vi "Intake Wheels Controller.vi"(8 "error in":errorcluster) -> ()   [LabVIEW 2017]
doc: "This VI executes continuously carrying out the current operation and responding to updates or new operations. It will often contain the timing or control code that is difficult to place directly in TeleOp. This VI generally opens all sensors and motors and isolates the rest of the robot code from knowing how the operations are carried out."
uses:
  <vilib>/Rock Robotics/WPI/Framework/Completion Status.ctl
  Intake Wheels Setpoints.ctl
  Intake Wheels Operations.ctl
  <vilib>/Rock Robotics/WPI/Solenoid/WPI_SolenoidValue.ctl
  <vilib>/Rock Robotics/WPI/Solenoid/WPI_SolenoidChannel.ctl
  Users/Public/Documents/Cross The Road Electronics/Phoenix-LabVIEW/Motor Controller/Controls/CTRE_Phoenix_MotorControl_ControlMode.ctl
  <vilib>/Rock Robotics/WPI/ThirdParty/Phoenix-LabVIEW/Motor Controller/Controls/CTRE_Phoenix_MotorControl_NeutralMode.ctl
  <vilib>/Rock Robotics/WPI/Solenoid/WPI_SolenoidOpenSingle.vi
  <vilib>/Rock Robotics/WPI/Solenoid/WPI_SolenoidSetEnum.vi
  <vilib>/Rock Robotics/Network Tables/NT Write Boolean.vi
panel:
  in  "Interactive Values":T1
  out "Current\nCmd":string
  in  "Buttons":cluster{"Execute Cmd":bool, "Abort Cmd":bool}
  out "Command Timing":cluster{"Start Time (ms)":u32, "Iterations":i32}
  out "Status":T3
  # "Tip: It may be helpful to observe inputs and sensor values.\nYou may also want to display tuning or debugging controls."
  # "Interactive Command: You may fill in the settings for a command\nand schedule it with the Execute button. You can observe and abort\nany command while fine tuning the code for the controller."
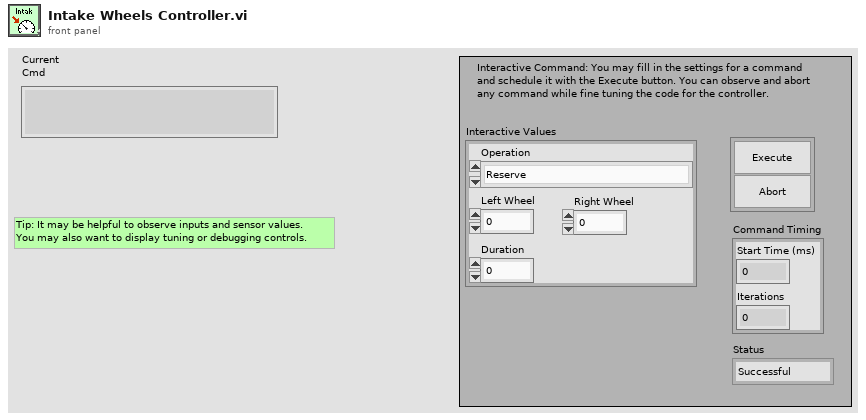
[diagram p1: front panel]
types:
  T1 = typedef "Intake Wheels Setpoints.ctl" = cluster{"Operation":T2, "Left Wheel":dbl, "Duration":dbl, "Right Wheel":dbl}
  T2 = typedef "Intake Wheels Operations.ctl" = enum16{"Reserve", "Read Current", "Immediate", "Intake Open", "Intake Close", "Wheels On"}
  T3 = typedef "Completion Status.ctl" = enum16{"Successful", "Aborted", "Incomplete"}
  T4 = typedef "CTRE_Phoenix_MotorControl_NeutralMode.ctl" = enum8{"EEPROMSetting", "Override to Coast", "Override to Brake"}
  T5 = typedef "CTRE_Phoenix_MotorControl_ControlMode.ctl" = u16
  T6 = typedef "WPI_SolenoidChannel.ctl" = enum8{"Solenoid 0", "Solenoid 1", "Solenoid 2", "Solenoid 3", "Solenoid 4", "Solenoid 5", "Solenoid 6", "Solenoid 7", "Invalid"}
  T7 = typedef "WPI_SolenoidValue.ctl" = enum16{"Off", "On", "Forward", "Reverse"}
  T8 = typedef "WPI_SolenoidDevRef.ctl" = cluster{"DevStatus":errorcluster, "Pneumatics Control Module":u8, "Forward Solenoid Channel":T6, "Reverse Solenoid Channel":T6}
  T9 = typedef "WPI_MotorControlDeviceRef.ctl" = cluster{"DeviceStatus":errorcluster, "Type":T10, "PWM":cluster{"PWM Channel":T11, "DeadBand":T12}, "CAN":cluster{"Device Number":u8, "SetOutput VI Ref":variant, "GetOutput VI Ref":variant, "Enable VI Ref":variant, "Disable VI Ref":variant, "Data":variant}, "Invert":bool, "DIO PWM":cluster{"PWM \"Enable\" Channel":T11, "DIOChannel":T13, "PWM Rate":dbl}}
  T10 = typedef "WPI_MotorControlType.ctl" = enum16{"PWM", "CAN", "DIO PWM"}
  T11 = typedef "FPGA_DIOPWMChannel.ctl" = enum8{"PWM 0", "PWM 1", "PWM 2", "PWM 3", "PWM 4", "PWM 5", "PWM 6", "PWM 7", "PWM 8", "PWM 9", "PWM MXP 0", "PWM MXP 1", "PWM MXP 2", "PWM MXP 3", "PWM MXP 4", "PWM MXP 5", "PWM MXP 6", "PWM MXP 7", "PWM MXP 8", "PWM MXP 9", "Invalid"}
  T12 = typedef "WPI_PWMDeadband.ctl" = cluster{"Name":string, "maxPositivePwm":i32, "minPositivePwm":i32, "centerPwm":i32, "maxNegativePwm":i32, "minNegativePwm":i32, "angularRange":u16}
  T13 = typedef "FPGA_DIOChannel.ctl" = enum8{"DIO 0", "DIO 1", "DIO 2", "DIO 3", "DIO 4", "DIO 5", "DIO 6", "DIO 7", "DIO 8", "DIO 9", "DIO MXP 0", "DIO MXP 1", "DIO MXP 2", "DIO MXP 3", "DIO MXP 4", "DIO MXP 5", "DIO MXP 6", "DIO MXP 7", "DIO MXP 8", "DIO MXP 9", "DIO MXP 10", "DIO MXP 11", "DIO MXP 12", "DIO MXP 13", "DIO MXP 14", "DIO MXP 15", "SPI Port CS1", "SPI Port CS2", "SPI Port CS3", "SPI Port MISO", "SPI Port MOSI", "Invalid"}
  T14 = typedef "Command Status Info.ctl" = cluster{"Name":string, "Status":T3, "notifier out":T15}
  T15 = typedef "Completion Notifier.ctl" = refnum<notifier>
  T16 = cluster{"Current Command":T1, "Command Timing":cluster{"Start Time (ms)":u32, "Iterations":i32}, "Command Arguments":cluster{"Command Info":T14, "Description":string, "Default Command":T1, "queue out":refnum<queue>, "Subsystem Name":string}}
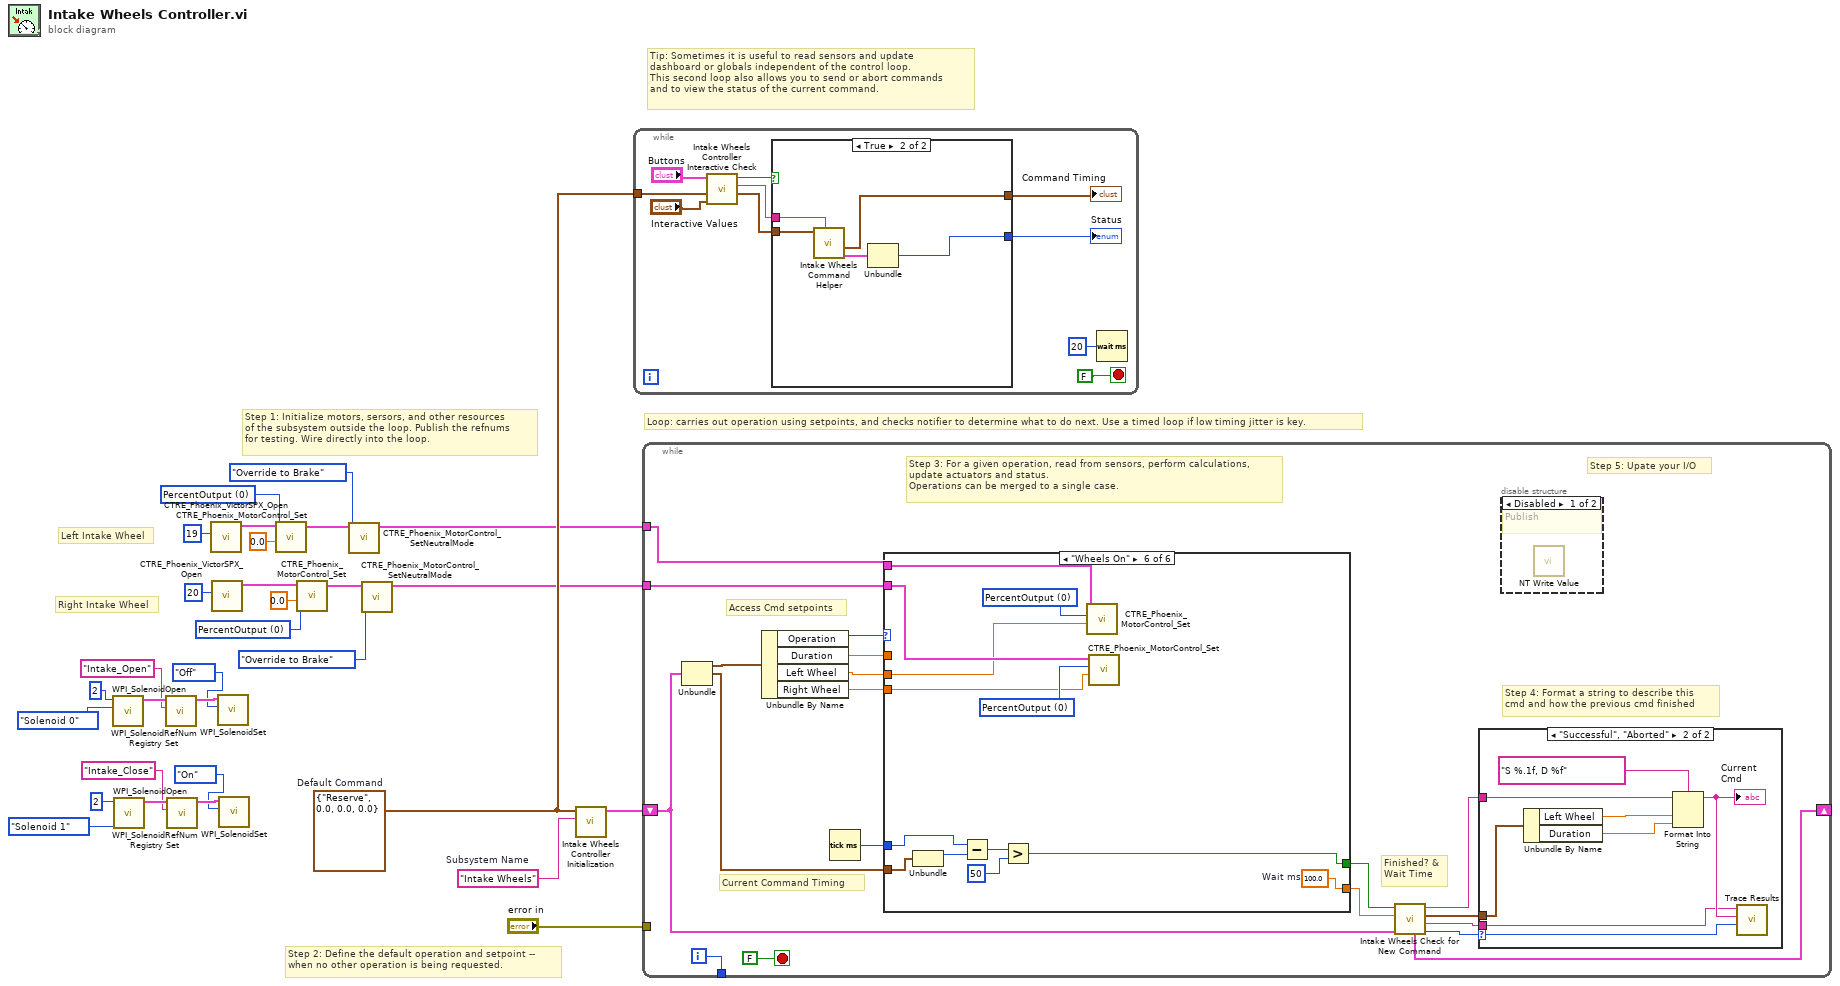
[diagram p0: block diagram]
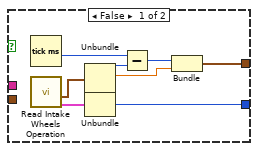
[diagram p2: hidden frame]
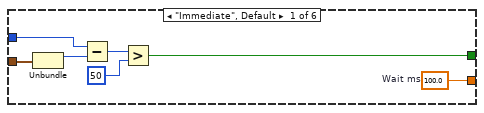
[diagram p5: hidden frame]
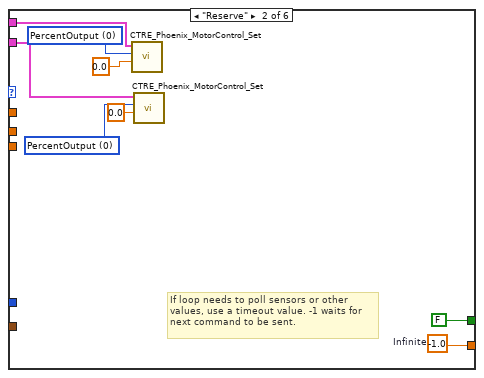
[diagram p6: hidden frame]
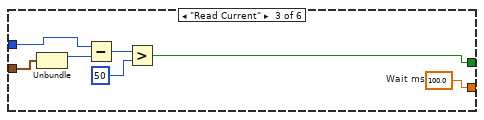
[diagram p7: hidden frame]
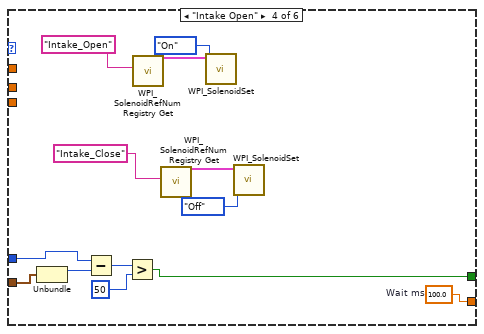
[diagram p8: hidden frame]
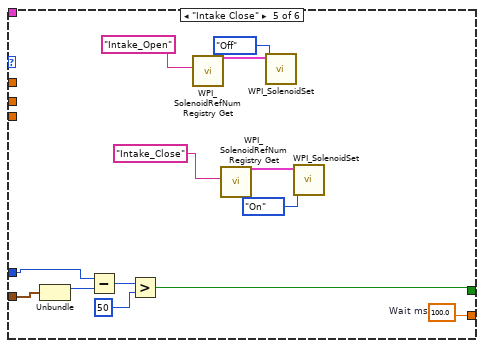
[diagram p9: hidden frame]
diagram:
  w10 = T5 0 items=["PercentOutput"=0, "Position"=1, "Velocity"=2, "Current"=3, "Follower"=5, "MotionProfile"=6, "MotionMagic"=7, "MotionMagicArc"=8, "MotionProfileArc"=10, "Disabled"=15] ("Control Mode")
  w11 = T5 0 items=["PercentOutput"=0, "Position"=1, "Velocity"=2, "Current"=3, "Follower"=5, "MotionProfile"=6, "MotionMagic"=7, "MotionMagicArc"=8, "MotionProfileArc"=10, "Disabled"=15] ("Control Mode")
  w27 = T1 {"Operation"=enum."Reserve", "Left Wheel"=0.0, "Duration"=0.0, "Right Wheel"=0.0}  # Default Command
  w28 = "Intake Wheels"  # Subsystem Name
  # "Right Intake Wheel"
  # "Left Intake Wheel"
  # "Tip: Sometimes it is useful to read sensors and update\ndashboard or globals independent of the control loop.\nThis second loop also allows you to send or abort commands\nand to view the status of the current command."
  # "Step 2: Define the default operation and setpoint --\nwhen no other operation is being requested."
  # "Step 1: Initialize motors, sersors, and other resources\nof the subsystem outside the loop. Publish the refnums\nfor testing. Wire directly into the loop."
  # "Loop: carries out operation using setpoints, and checks notifier to determine what to do next. Use a timed loop if low timing jitter is key."
  n1 = call-poly <vilib>:"WPI_SolenoidOpen.vi"("Solenoid Channel"=WPI_SolenoidChannel."Solenoid 0", "Pneumatics Control Module (0)"=u8 2) -> ("SolenoidDevRef"=w26:T8)  [unwired: 8 in, 1 out]
  n2 = call-poly <vilib>:"WPI_SolenoidOpen.vi"("Solenoid Channel"=WPI_SolenoidChannel."Solenoid 1", "Pneumatics Control Module (0)"=u8 2) -> ("SolenoidDevRef"=w21:T8)  [unwired: 8 in, 1 out]
  n3 = call <vilib>:"WPI_SolenoidRefNum Registry Set.vi"("refnum name"="Intake_Open", "SolenoidDevRef"=w26) -> ("SolenoidDevRef"=w25:T8)  [unwired: 8 in, 1 out]
  n4 = call <vilib>:"WPI_SolenoidRefNum Registry Set.vi"("refnum name"="Intake_Close", "SolenoidDevRef"=w21) -> ("SolenoidDevRef"=w20:T8)  [unwired: 8 in, 1 out]
  n5 = call <vilib>:"CTRE_Phoenix_VictorSPX_Open.vi"("Device Number"=u8 19) -> ("CAN Talon SRX Ref"=w12:T9)  [unwired: 9 in, 1 out]
  n6 = call <vilib>:"CTRE_Phoenix_VictorSPX_Open.vi"("Device Number"=u8 20) -> ("CAN Talon SRX Ref"=w9:T9)  [unwired: 9 in, 1 out]
  n7 = call-poly <vilib>:"WPI_SolenoidSet.vi"("Value"=WPI_SolenoidValue."Off", "SolenoidDevRef"=w25) -> ()  [unwired: 8 in, 2 out]
  n8 = call-poly <vilib>:"WPI_SolenoidSet.vi"("Value"=WPI_SolenoidValue."On", "SolenoidDevRef"=w20) -> ()  [unwired: 8 in, 2 out]
  n9 = call <vilib>:"CTRE_Phoenix_MotorControl_Set.vi"("Output"=0.0, "Control Mode"=w11, "PhoenixMotorControlDevRef"=w12) -> ("PhoenixMotorControlDevRef"=w8:T9)  [unwired: 7 in, 1 out]
  n10 = call <vilib>:"CTRE_Phoenix_MotorControl_Set.vi"("Output"=0.0, "Control Mode"=w10, "PhoenixMotorControlDevRef"=w9) -> ("PhoenixMotorControlDevRef"=w6:T9)  [unwired: 7 in, 1 out]
  n11 = call <vilib>:"CTRE_Phoenix_MotorControl_SetNeutralMode.vi"("Motor Control Neutral Mode"=CTRE_Phoenix_MotorControl_NeutralMode."Override to Brake", "PhoenixMotorControlDevRef"=w8) -> ("PhoenixMotorControlDevRef"=w2:T9)  [unwired: 8 in, 1 out]
  n12 = call <vilib>:"CTRE_Phoenix_MotorControl_SetNeutralMode.vi"("Motor Control Neutral Mode"=CTRE_Phoenix_MotorControl_NeutralMode."Override to Brake", "PhoenixMotorControlDevRef"=w6) -> ("PhoenixMotorControlDevRef"=w1:T9)  [unwired: 8 in, 1 out]
  n13 = call "Intake Wheels Controller Initialization.vi"("Subsystem Name"=w28, "Default Command"=w27) -> ("Current Command"=w29:T16)  [unwired: 9 in]
  n14 = while {
    tunnel: w27 -> [w37]
    stop <- FALSE stop-if-true
    n15 = call "Intake Wheels Controller Interactive Check.vi"("Interactive Command in"="Interactive Values", "Default Command"=w37, "Buttons"="Buttons") -> ("Interactive Command out"=w34:T1, "Trace String"=w35:string, "Schedule"=w36:bool)  [unwired: 6 in]
    n16 = case shown="True" w36 {
      tunnel: [w48 w53] -> w33
      tunnel: w34 -> [_ w51]
      tunnel: [w44 w49] -> w32
      tunnel: w35 -> [_ w52]
      frame False {
        n17 = Tick Count (ms)() -> (millisecond timer value=w43:u32)
        n18 = call "Read Intake Wheels Operation.vi"() -> ("Command Info"=w41:T14, "SubSystem Data"=w42:T1)  [unwired: 9 in, 1 out]
        n19 = Unbundle(w42) -> ("Operation"=w47:T2, "Left Wheel"=w45:dbl)  [unwired: 2 out]
        n20 = Unbundle(w41) -> ("Status"=w48:T3)  [unwired: 2 out]
        n21 = Subtract(x=w43, y=w47) -> (x-y=w46:u32)
        n22 = Bundle(w46, "Left Wheel"=w45) -> (w44:cluster{u32, "Left Wheel":dbl})  [unwired: 1 in]
      }
      frame True {
        n23 = call "Intake Wheels Command Helper.vi"("Description"=w52, "SubSystem Data"=w51) -> ("Command Info Out"=w50:T14, "Command Timing"=w49:cluster{"Start Time (ms)":u32, "Iterations":i32})  [unwired: 7 in, 1 out]
        n24 = Unbundle(w50) -> ("Status"=w53:T3)  [unwired: 2 out]
      }
    }
    "Status" <- w33
    "Command Timing" <- w32
    n25 = Wait (ms)(milliseconds to wait=u32 20) -> ()  [unwired: 1 out]
  }
  n26 = while {
    shift-right: [w64] -> _
    shift-left: w29 -> [w57]
    tunnel: [w71] -> _
    tunnel: "error in" -> [_]
    tunnel: w2 -> [w56]
    tunnel: w1 -> [w55]
    i -> [w71]
    stop <- FALSE stop-if-true
    # "Step 5: Upate your I/O"
    # "Step 4: Format a string to describe this\ncmd and how the previous cmd finished"
    # "Current Command Timing"
    # "Access Cmd setpoints"
    # "Finished? &\nWait Time"
    # "Step 3: For a given operation, read from sensors, perform calculations,\nupdate actuators and status.\nOperations can be merged to a single case."
    n27 = Unbundle(w57) -> ("Current Command"=w70:T1, "Command Timing"=w66:cluster{"Start Time (ms)":u32, "Iterations":i32})  [unwired: 1 out]
    n28 = Unbundle By Name(w70) -> ("Operation"=w69:T2, "Duration"=w68:dbl, "Left Wheel"=w65:dbl, "Right Wheel"=w54:dbl)
    n29 = Tick Count (ms)() -> (millisecond timer value=w67:u32)
    n30 = case shown="\"Wheels On\"" w69 {
      tunnel: [w87 w95 w97 w110 w122 w135] -> w62
      tunnel: [w81 FALSE ("ignore previous (F)") w96 w109 w123 w136] -> w63
      tunnel: w66 -> [w83 _ w98 w111 w124 w137]
      tunnel: w68 -> [_ _ _ _ _ _]
      tunnel: w67 -> [w82 _ w99 w112 w125 w138]
      tunnel: w65 -> [_ _ _ _ _ w130]
      tunnel: w56 -> [_ w93 _ _ _ w132]
      tunnel: w55 -> [_ w92 _ _ _ w131]
      tunnel: w54 -> [_ _ _ _ _ w129]
      frame "Immediate", Default {
        w87 = 100.0  # Wait ms
        n31 = Unbundle(w83) -> ("Start Time (ms)"=w86:u32)  [unwired: 1 out]
        n32 = Subtract(x=w82, y=w86) -> (x-y=w85:u32)
        n33 = Greater?(x=w85, y=u8 50 ("Left Motor")) -> (0:w81:bool)
      }
      frame "Reserve" {
        w90 = T5 0 items=["PercentOutput"=0, "Position"=1, "Velocity"=2, "Current"=3, "Follower"=5, "MotionProfile"=6, "MotionMagic"=7, "MotionMagicArc"=8, "MotionProfileArc"=10, "Disabled"=15] ("Control Mode")
        w91 = T5 0 items=["PercentOutput"=0, "Position"=1, "Velocity"=2, "Current"=3, "Follower"=5, "MotionProfile"=6, "MotionMagic"=7, "MotionMagicArc"=8, "MotionProfileArc"=10, "Disabled"=15] ("Control Mode")
        w95 = -1.0  # Infinite
        # "If loop needs to poll sensors or other\nvalues, use a timeout value. -1 waits for\nnext command to be sent."
        n34 = call <vilib>:"CTRE_Phoenix_MotorControl_Set.vi"("Output"=0.0, "Control Mode"=w91, "PhoenixMotorControlDevRef"=w93) -> ()  [unwired: 7 in, 2 out]
        n35 = call <vilib>:"CTRE_Phoenix_MotorControl_Set.vi"("Output"=0.0, "Control Mode"=w90, "PhoenixMotorControlDevRef"=w92) -> ()  [unwired: 7 in, 2 out]
      }
      frame "Read Current" {
        w97 = 100.0  # Wait ms
        n36 = Unbundle(w98) -> ("Start Time (ms)"=w102:u32)  [unwired: 1 out]
        n37 = Subtract(x=w99, y=w102) -> (x-y=w101:u32)
        n38 = Greater?(x=w101, y=u8 50 ("Left Motor")) -> (0:w96:bool)
      }
      frame "Intake Open" {
        w110 = 100.0  # Wait ms
        n39 = Unbundle(w111) -> ("Start Time (ms)"=w114:u32)  [unwired: 1 out]
        n40 = Subtract(x=w112, y=w114) -> (x-y=w115:u32)
        n41 = Greater?(x=w115, y=u8 50 ("Left Motor")) -> (0:w109:bool)
        n42 = call <vilib>:"WPI_SolenoidRefNum Registry Get.vi"("refnum name"="Intake_Open") -> ("SolenoidDevRef"=w108:T8)  [unwired: 9 in, 1 out]
        n43 = call <vilib>:"WPI_SolenoidRefNum Registry Get.vi"("refnum name"="Intake_Close") -> ("SolenoidDevRef"=w106:T8)  [unwired: 9 in, 1 out]
        n44 = call-poly <vilib>:"WPI_SolenoidSet.vi"("Value"=WPI_SolenoidValue."On", "SolenoidDevRef"=w108) -> ()  [unwired: 8 in, 2 out]
        n45 = call-poly <vilib>:"WPI_SolenoidSet.vi"("Value"=WPI_SolenoidValue."Off", "SolenoidDevRef"=w106) -> ()  [unwired: 8 in, 2 out]
      }
      frame "Intake Close" {
        w122 = 100.0  # Wait ms
        n46 = Unbundle(w124) -> ("Start Time (ms)"=w127:u32)  [unwired: 1 out]
        n47 = Subtract(x=w125, y=w127) -> (x-y=w128:u32)
        n48 = Greater?(x=w128, y=u8 50 ("Left Motor")) -> (0:w123:bool)
        n49 = call <vilib>:"WPI_SolenoidRefNum Registry Get.vi"("refnum name"="Intake_Open") -> ("SolenoidDevRef"=w121:T8)  [unwired: 9 in, 1 out]
        n50 = call <vilib>:"WPI_SolenoidRefNum Registry Get.vi"("refnum name"="Intake_Close") -> ("SolenoidDevRef"=w119:T8)  [unwired: 9 in, 1 out]
        n51 = call-poly <vilib>:"WPI_SolenoidSet.vi"("Value"=WPI_SolenoidValue."Off", "SolenoidDevRef"=w121) -> ()  [unwired: 8 in, 2 out]
        n52 = call-poly <vilib>:"WPI_SolenoidSet.vi"("Value"=WPI_SolenoidValue."On", "SolenoidDevRef"=w119) -> ()  [unwired: 8 in, 2 out]
      }
      frame "Wheels On" {
        w133 = T5 0 items=["PercentOutput"=0, "Position"=1, "Velocity"=2, "Current"=3, "Follower"=5, "MotionProfile"=6, "MotionMagic"=7, "MotionMagicArc"=8, "MotionProfileArc"=10, "Disabled"=15] ("Control Mode")
        w134 = T5 0 items=["PercentOutput"=0, "Position"=1, "Velocity"=2, "Current"=3, "Follower"=5, "MotionProfile"=6, "MotionMagic"=7, "MotionMagicArc"=8, "MotionProfileArc"=10, "Disabled"=15] ("Control Mode")
        w135 = 100.0  # Wait ms
        n53 = Unbundle(w137) -> ("Start Time (ms)"=w141:u32)  [unwired: 1 out]
        n54 = Subtract(x=w138, y=w141) -> (x-y=w140:u32)
        n55 = Greater?(x=w140, y=u8 50 ("Left Motor")) -> (0:w136:bool)
        n56 = call <vilib>:"CTRE_Phoenix_MotorControl_Set.vi"("Output"=w130, "Control Mode"=w134, "PhoenixMotorControlDevRef"=w132) -> ()  [unwired: 7 in, 2 out]
        n57 = call <vilib>:"CTRE_Phoenix_MotorControl_Set.vi"("Output"=w129, "Control Mode"=w133, "PhoenixMotorControlDevRef"=w131) -> ()  [unwired: 7 in, 2 out]
      }
    }
    n58 = call "Intake Wheels Check for New Command.vi"("Current Command"=w57, "Wait time (ms)"=w62, "Finished?"=w63) -> ("Completion"=w58:T3, "Subsystem Name"=w59:string, "Current Command"=w60:T1, "Initial Trace String"=w61:string, "NextCommand"=w64:T16)  [unwired: 4 in]
    n59 = case shown="\"Successful\", \"Aborted\"" w58 {
      selector: w58 -> [_ w80]
      tunnel: w61 -> [_ w76]
      tunnel: w60 -> [_ w77]
      tunnel: w59 -> [_ w73]
      frame "Incomplete", Default {
        # "Continuing current command"
      }
      frame "Successful", "Aborted" {
        # "Report and setup for next command"
        n60 = Unbundle By Name(w77) -> ("Left Wheel"=w79:dbl, "Duration"=w74:dbl)
        n61 = Format Into String(format string="S %.1f, D %f", initial string=w76, w79, w74) -> (resulting string=w75:string)  [unwired: 1 in, 1 out]
        "Current\nCmd" <- w75
        n62 = call <vilib>:"Trace Results.vi"("Status of previous command"=w80, "Description"=w75, "Subsystem"=w73) -> ()  [unwired: 9 in]
      }
    }
    n63 = disable-structure shown="Disabled" {
      frame Disabled {
        # "Publish"
        n64 = call-poly <vilib>:"NT Write Value.vi"() -> ()  [unwired: 11 in, 1 out]
      }
      frame Enabled {
      }
    }
  }
